vi "Percentage.vi"(2 "Input Array":i32[](array[numeric]), 5 "Thresholds":dbl[](array[numeric])) -> (14 "Cat 1":dbl, 15 "Cat 2":dbl, 16 "Cat 3":dbl, 17 "Cat 4":dbl, 18 "Cat 5":dbl, 19 "Cat 6":dbl)   [LabVIEW 2020, in "Parameters Lib.lvlib"]
uses:
  Parameters Lib.lvlib
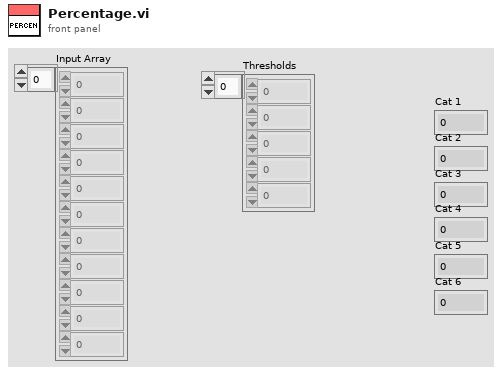
[diagram p1: front panel]
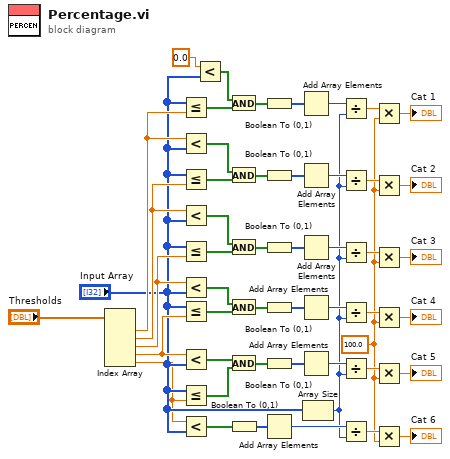
[diagram p0: block diagram]
diagram:
  w7 = 100.0 ("y")
  n1 = Index Array(array="Thresholds") -> (element #1=w48:dbl, element #2=w47:dbl, element #3=w46:dbl, element #4=w45:dbl, element #5=w43:dbl)  [unwired: 5 in]
  n2 = Less Or Equal?(x="Input Array", y=w48) -> (x <= y?=w41:bool[])
  n3 = Less?(x=w48, y="Input Array") -> (x < y?=w39:bool[])
  n4 = Less Or Equal?(x="Input Array", y=w47) -> (x <= y?=w40:bool[])
  n5 = Less?(x=w47, y="Input Array") -> (x < y?=w37:bool[])
  n6 = Less Or Equal?(x="Input Array", y=w46) -> (x <= y?=w38:bool[])
  n7 = Less?(x=w46, y="Input Array") -> (x < y?=w35:bool[])
  n8 = Less Or Equal?(x="Input Array", y=w45) -> (x <= y?=w36:bool[])
  n9 = Less?(x=w45, y="Input Array") -> (x < y?=w34:bool[])
  n10 = Less Or Equal?(x="Input Array", y=w43) -> (x <= y?=w33:bool[])
  n11 = Less?(x=w43, y="Input Array") -> (x < y?=w22:bool[])
  n12 = Less?(x=0.0, y="Input Array") -> (x < y?=w42:bool[])
  n13 = And(x=w42, y=w41) -> (x .and. y?=w32:bool[])
  n14 = And(x=w39, y=w40) -> (x .and. y?=w31:bool[])
  n15 = And(x=w37, y=w38) -> (x .and. y?=w30:bool[])
  n16 = And(x=w35, y=w36) -> (x .and. y?=w29:bool[])
  n17 = And(x=w34, y=w33) -> (x .and. y?=w28:bool[])
  n18 = Boolean To (0,1)(Boolean=w22) -> (0, 1=w21:i16[])
  n19 = Boolean To (0,1)(Boolean=w32) -> (0, 1=w27:i16[])
  n20 = Boolean To (0,1)(Boolean=w31) -> (0, 1=w26:i16[])
  n21 = Boolean To (0,1)(Boolean=w30) -> (0, 1=w25:i16[])
  n22 = Boolean To (0,1)(Boolean=w29) -> (0, 1=w24:i16[])
  n23 = Boolean To (0,1)(Boolean=w28) -> (0, 1=w23:i16[])
  n24 = Add Array Elements(numeric array=w21) -> (sum=w15:i16)
  n25 = Add Array Elements(numeric array=w27) -> (sum=w20:i16)
  n26 = Add Array Elements(numeric array=w26) -> (sum=w19:i16)
  n27 = Add Array Elements(numeric array=w25) -> (sum=w18:i16)
  n28 = Add Array Elements(numeric array=w24) -> (sum=w17:i16)
  n29 = Add Array Elements(numeric array=w23) -> (sum=w16:i16)
  n30 = Array Size(array="Input Array") -> (size(s)=w14:i32)
  n31 = Divide(x=w20, y=w14) -> (x/y=w8:dbl)
  n32 = Divide(x=w19, y=w14) -> (x/y=w9:dbl)
  n33 = Divide(x=w18, y=w14) -> (x/y=w10:dbl)
  n34 = Divide(x=w17, y=w14) -> (x/y=w11:dbl)
  n35 = Divide(x=w16, y=w14) -> (x/y=w12:dbl)
  n36 = Divide(x=w15, y=w14) -> (x/y=w13:dbl)
  n37 = Multiply(x=w8, y=w7) -> (x*y=→"Cat 1":dbl)
  n38 = Multiply(x=w9, y=w7) -> (x*y=→"Cat 2":dbl)
  n39 = Multiply(x=w10, y=w7) -> (x*y=→"Cat 3":dbl)
  n40 = Multiply(x=w11, y=w7) -> (x*y=→"Cat 4":dbl)
  n41 = Multiply(x=w12, y=w7) -> (x*y=→"Cat 5":dbl)
  n42 = Multiply(x=w13, y=w7) -> (x*y=→"Cat 6":dbl)
